vi "Set as Input.vi"(8 "error in (no error)":errorcluster, 10 "Direction":bool, 11 "Channel Ref in":T1 format="%.0x") -> (0 "error out":errorcluster, 3 "Channel Ref out":T1=18446744073709551615 format="%.0x")   [LabVIEW 2019, in "Modbus Master System Explorer.lvlib"]
uses:
  Modbus Master System Explorer.lvlib
  <vilib>/NI VeriStand/Custom Device API/Custom Device Item Ref.ctl
  <vilib>/NI VeriStand/Custom Device API/Custom Device Channel Type.ctl
  <vilib>/NI VeriStand/Custom Device API/Custom Device API.lvlib
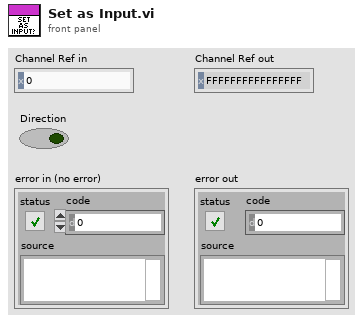
[diagram p1: front panel]
types:
  T1 = typedef "Custom Device API.lvlib/Custom Device Item Ref.ctl" = u64
  T2 = typedef "Custom Device API.lvlib/Custom Device Channel Type.ctl" = enum16{"Input", "Output"}
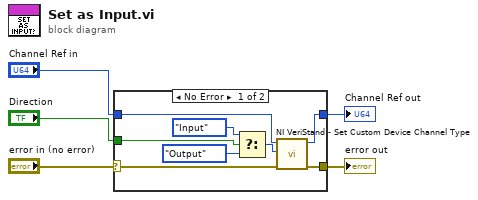
[diagram p0: block diagram]
diagram:
  n1 = case shown="No Error" "error in (no error)" {
    selector: "error in (no error)" -> [w12 w15]
    tunnel: [w13 w15] -> w5
    tunnel: "Direction" -> [w8 _]
    tunnel: "Channel Ref in" -> [w7 w14]
    tunnel: [w6 w14] -> w1
    frame No Error {
      n2 = Select(t=Custom_Device_Channel_Type."Input" ("Type"), s=w8, f=Custom_Device_Channel_Type."Output") -> (s? t:f=w11:T2)
      n3 = call <vilib>:"NI VeriStand - Set Custom Device Channel Type.vi"("error in (no error)"=w12, "Type"=w11, "Channel Ref in"=w7) -> ("error out"=w13:errorcluster, "Channel Ref out"=w6:T1)  [unwired: 7 in]
    }
    frame Error {
    }
  }
  "error out" <- w5
  "Channel Ref out" <- w1
